vi "Format StartInstancesResult_LVXML_State.vi"(8 "error in (no error)":errorcluster, 10 "State Tag":string, 11 "valueXmlData":T2) -> (0 "error out":errorcluster, 2 "State.name":string, 3 "State.code":i16)   [LabVIEW 2014, in "AWS_EC2.lvlib" / "AWS_EC2.lvclass"]
uses:
  AWS_EC2.lvclass
  lv-xml-parser/r0/trunk/VI Source/EventType.ctl
  lv-xml-parser/r0/trunk/VI Source/LV XML Parser.lvlib
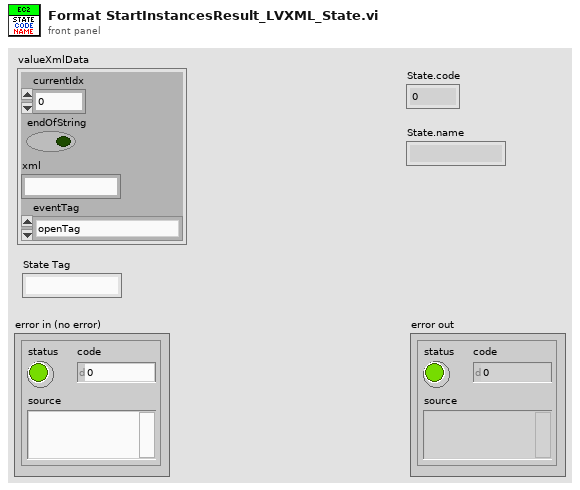
[diagram p1: front panel]
types:
  T1 = typedef "LV XML Parser.lvlib/EventType.ctl" = enum16{"openTag", "endOpenTag", "closeTag", "comment", "endComment", "endOfFile", "attribute", "startXml"}
  T2 = cluster{"currentIdx":i32, "endOfString":bool, "xml":string, "eventTag":T1}
  T3 = cluster{"namespaceUri":string, "localName":string}
  T4 = cluster{"Attributes":cluster{"localName":string, "namespaceUri":string, "value":string}[], "localName":string, "namespaceUri":string, "valueXmlData":cluster{"currentIdx":i32, "endOfString":bool, "xml":string, "eventTag":T1}}[]
  T5 = cluster{"Attributes":cluster{"localName":string, "namespaceUri":string, "value":string}[], "localName":string, "namespaceUri":string, "valueXmlData":cluster{"currentIdx":i32, "endOfString":bool, "xml":string, "eventTag":T1}}
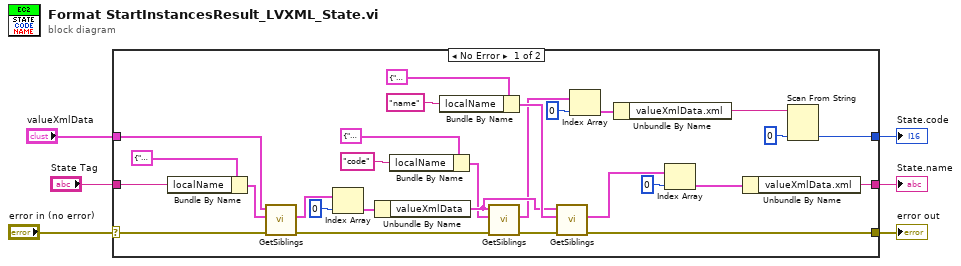
[diagram p0: block diagram]
diagram:
  n1 = case shown="No Error" "error in (no error)" {
    selector: "error in (no error)" -> [w10 w35]
    tunnel: "valueXmlData" -> [w34 _]
    tunnel: [w33 _] -> w5
    tunnel: [w25 _] -> w4
    tunnel: "State Tag" -> [w12 _]
    tunnel: [w7 w35] -> w2
    frame No Error {
      n2 = Bundle By Name(cluster=T3 {"namespaceUri"="", "localName"=""} ("limitToTag"), "localName"=w12) -> (w13:T3)
      n3 = call "GetSiblings.vi"("error in (no error)"=w10, "limitToTag"=w13, "xmlData"=w34) -> ("error out"=w9:errorcluster, "Siblings"=w18:T4)  [unwired: 7 in]
      n4 = Index Array(array=w18, index=0) -> (element=w19:T5)
      n5 = Unbundle By Name(w19) -> ("valueXmlData"=w30:T2)
      n6 = Bundle By Name(cluster=T3 {"namespaceUri"="", "localName"=""} ("limitToTag"), "localName"="code" ("Tag name")) -> (w20:T3)
      n7 = Bundle By Name(cluster=T3 {"namespaceUri"="", "localName"=""} ("limitToTag"), "localName"="name" ("Tag name")) -> (w32:T3)
      n8 = call "GetSiblings.vi"("error in (no error)"=w9, "limitToTag"=w20, "xmlData"=w30) -> ("error out"=w8:errorcluster, "Siblings"=w23:T4)  [unwired: 7 in]
      n9 = call "GetSiblings.vi"("error in (no error)"=w8, "limitToTag"=w32, "xmlData"=w30) -> ("error out"=w7:errorcluster, "Siblings"=w31:T4)  [unwired: 7 in]
      n10 = Index Array(array=w23, index=0) -> (element=w21:T5)
      n11 = Unbundle By Name(w21) -> ("valueXmlData.xml"=w24:string)
      n12 = Index Array(array=w31, index=0) -> (element=w27:T5)
      n13 = Unbundle By Name(w27) -> ("valueXmlData.xml"=w33:string)
      n14 = Scan From String(input string=w24, default 1=i16 0 ("currentState.code")) -> (output 1=w25:i16)  [unwired: 3 in, 3 out]
    }
    frame Error {
    }
  }
  "State.name" <- w5
  "State.code" <- w4
  "error out" <- w2
